vi "test-sync singleline loop.vi"(8 "error in (no error)":errorcluster, 11 "TestCase in":refnum<class "testcase-csm loop support.lvclass">) -> (0 "error out":errorcluster, 3 "TestCase out":refnum<class "testcase-csm loop support.lvclass">)   [LabVIEW 2017, in "testcase-csm loop support.lvclass"]
uses:
  testcase-csm loop support.lvclass
  56d4bdba-c2f1-4b55-add1-7a078de9da03.vi
  ea54eaf7-6c78-4206-8259-080cdfbb85de.vi
  src/user.lib/_NEVSTOP/Communicable State Machine(CSM)/AdvanceAPI/CSM - Revert Arguments-Safe String.vi
  src/user.lib/_NEVSTOP/Communicable State Machine(CSM)/_Shared/Trim Single-line Text.vi
  src/user.lib/_NEVSTOP/Communicable State Machine(CSM)/AdvanceAPI/CSM - Make String Arguments Safe.vi
  src/user.lib/_NEVSTOP/Communicable State Machine(CSM)/AdvanceAPI/CSM - Break Down Multiple States String.vi
  src/user.lib/_NEVSTOP/Communicable State Machine(CSM)/AdvanceAPI/CSM - Compact Multiple States.vi
  src/user.lib/_NEVSTOP/Communicable State Machine(CSM)/AdvanceAPI/CSM - Keywords.vi
  <vilib>/addons/_JKI Toolkits/VI Tester/TestCase.llb/TestCase.lvclass
  src/user.lib/_NEVSTOP/Communicable State Machine(CSM)/Communicable State Machine.lvlib
  src/user.lib/_NEVSTOP/Communicable State Machine(CSM)/addons/Loop-Support/CSM Loop Support.lvlib
  C:/Program Files (x86)/National Instruments/LabVIEW 2017/vi.lib/addons/_JKI Toolkits/VI Tester/TestCase.llb/TestCase.lvclass
panel:
  out "State History":string
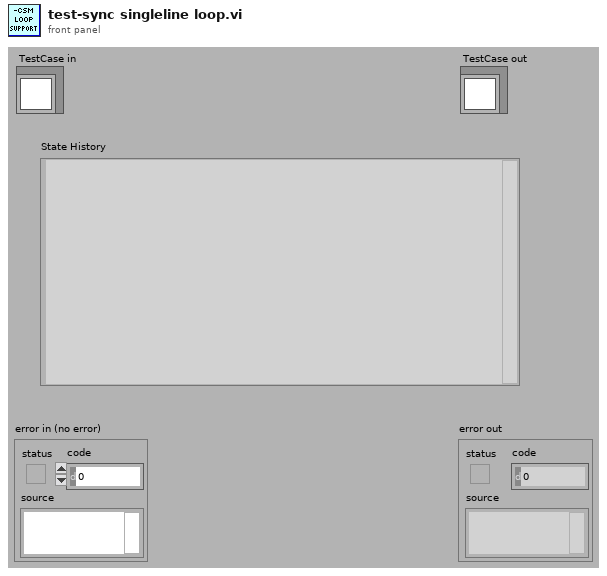
[diagram p1: front panel]
types:
  T1 = enum32{"Invalid", "Standard", "Closed", "Hidden", "Minimized", "Maximized"}
  T2 = enum32{"invalid app kind", "Development System", "Run Time System", "Student Edition", "Embedded LabVIEW", "Evaluation", "Custom"}
  T3 = typedef "Communicable State Machine.lvlib/_CSM_Response Source Message.ctl" = cluster{"‘State":string, "’Arguments":string, "’Error":errorcluster}
  T4 = cluster{"Current VI Reference":refnum<vi>, "Close Panel on Exit?":bool}
  T5 = cluster{"Core":cluster{"Current VI Reference":refnum<vi>, "Close Panel on Exit?":bool}, "diff":dbl, "time":timestamp}
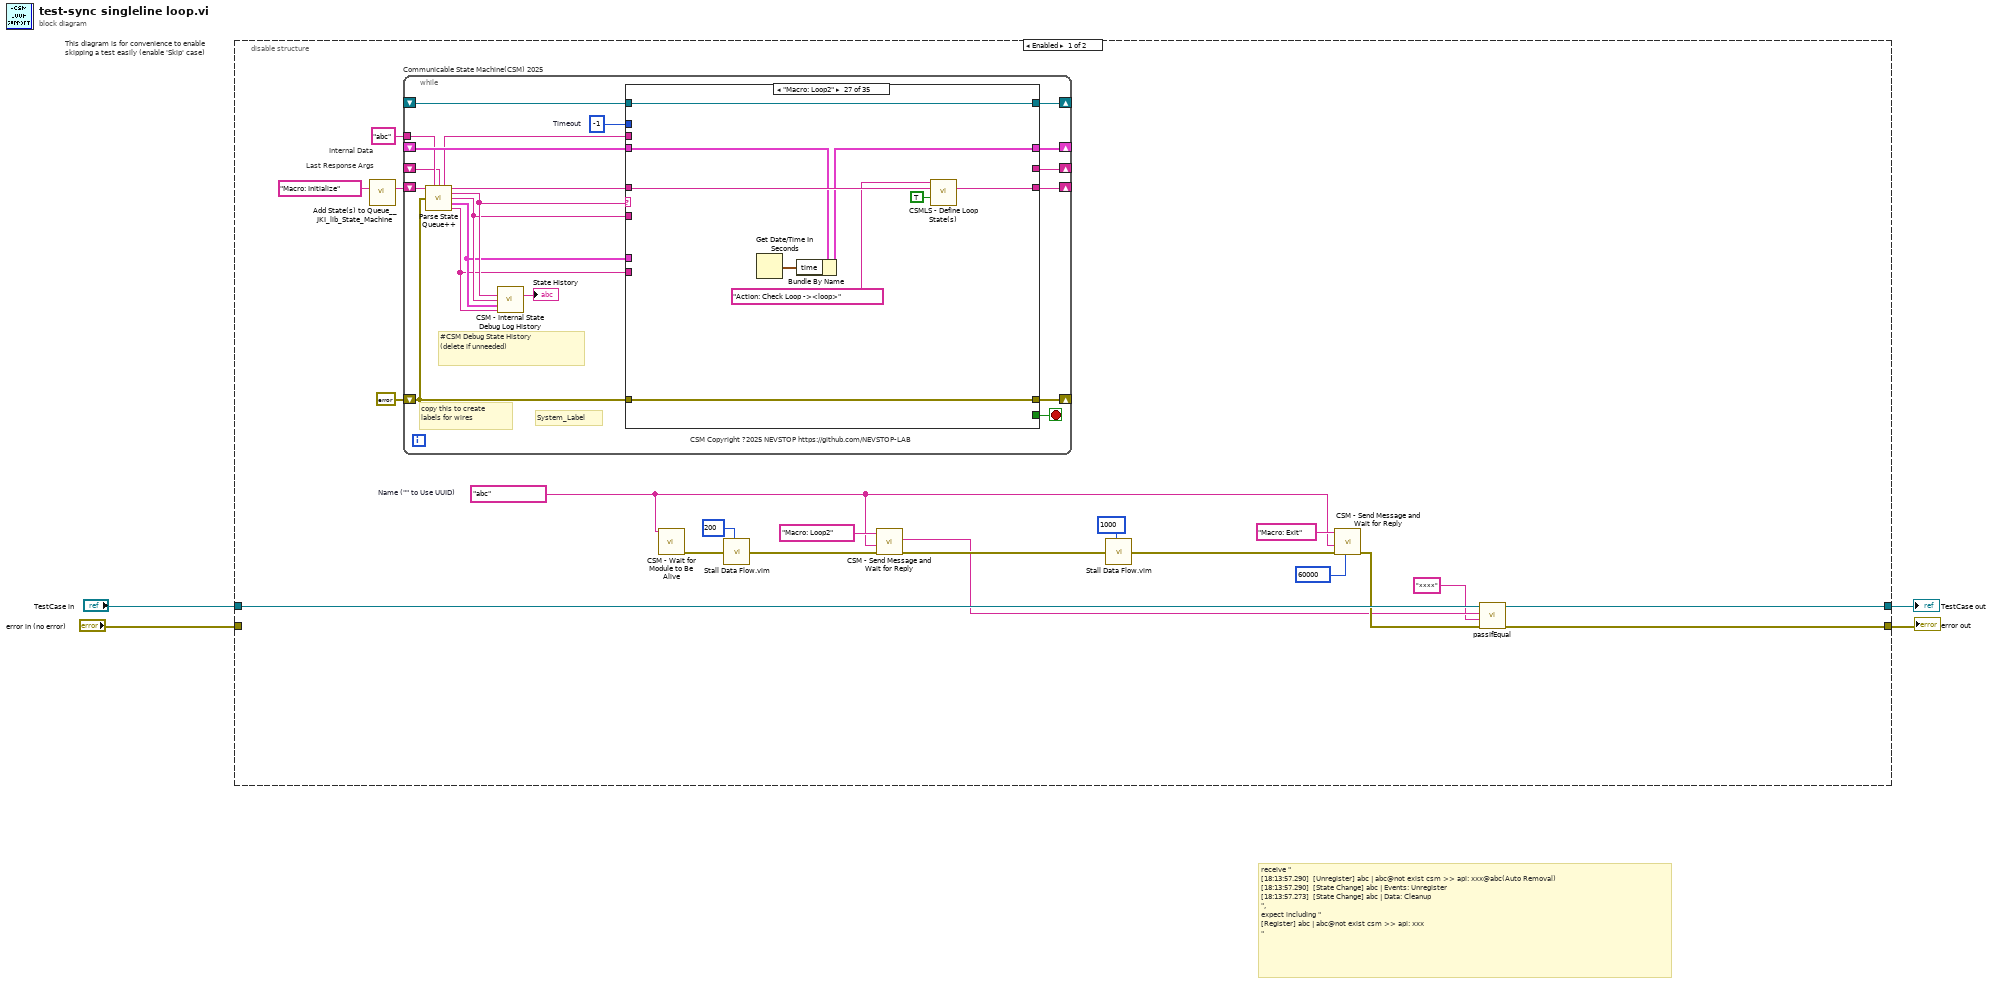
[diagram p0: block diagram]
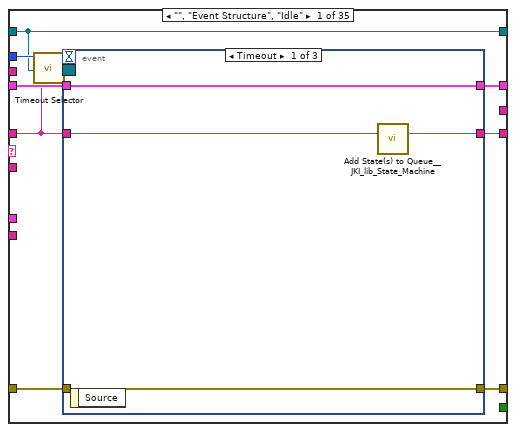
[diagram p2: hidden frame]
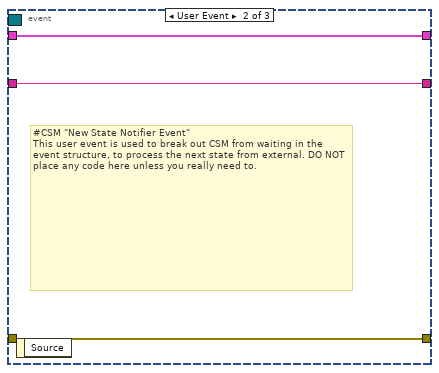
[diagram p3: hidden frame]
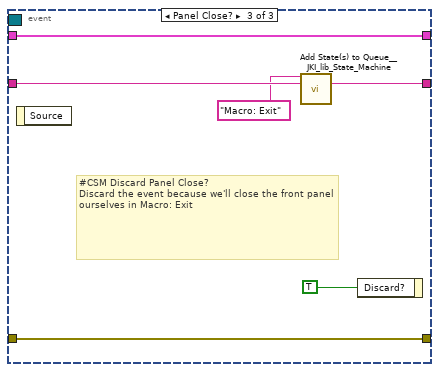
[diagram p4: hidden frame]
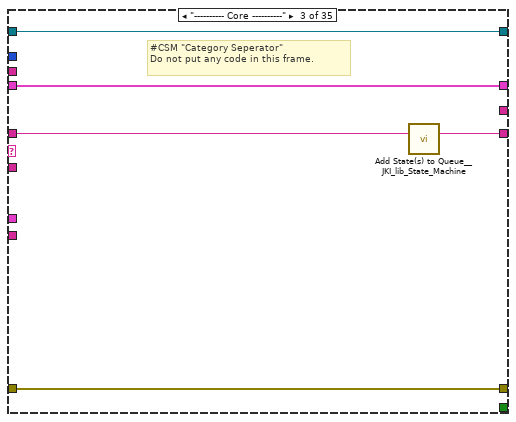
[diagram p6: hidden frame]
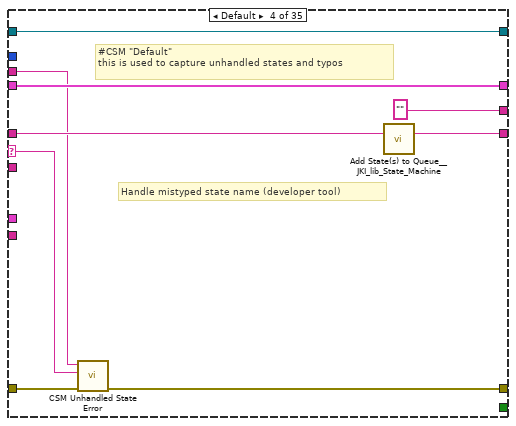
[diagram p7: hidden frame]
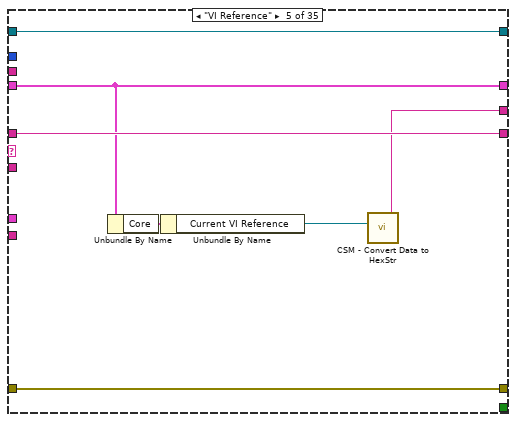
[diagram p8: hidden frame]
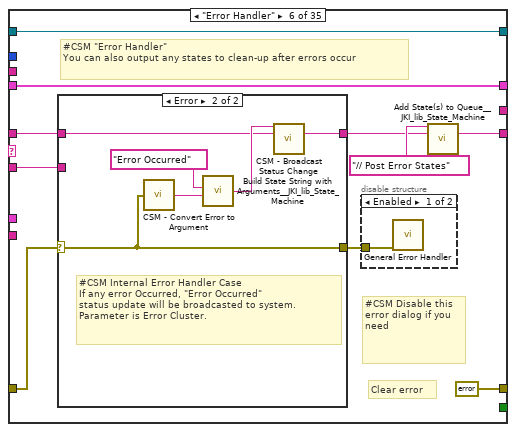
[diagram p9: hidden frame]
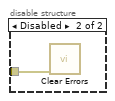
[diagram p10: hidden frame]
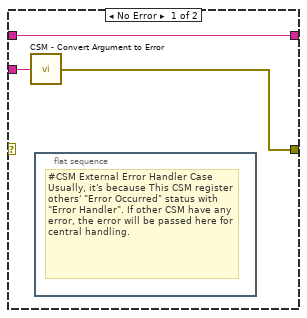
[diagram p11: hidden frame]
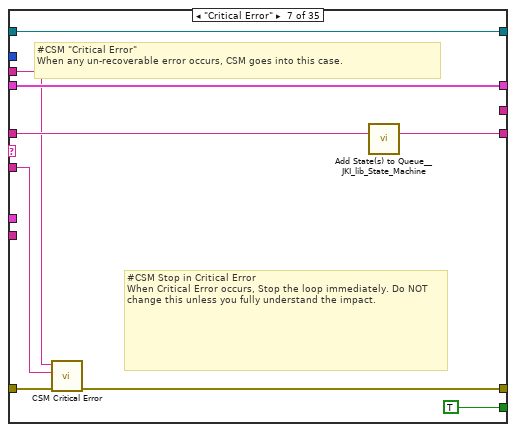
[diagram p12: hidden frame]
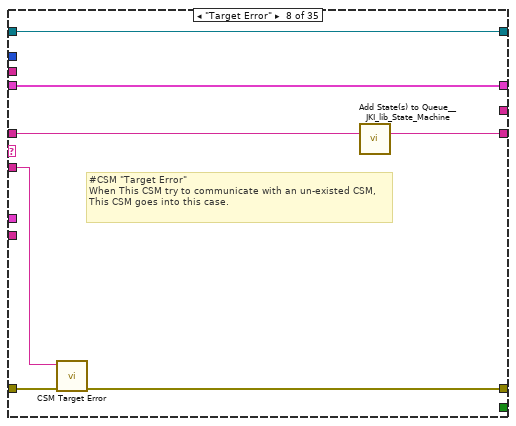
[diagram p13: hidden frame]
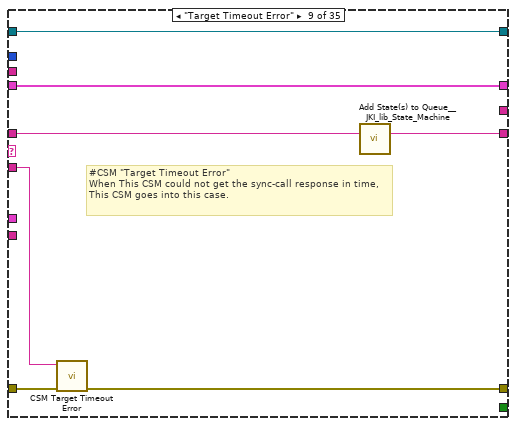
[diagram p14: hidden frame]
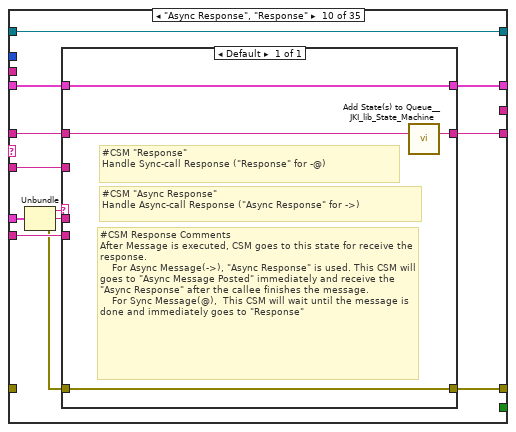
[diagram p15: hidden frame]
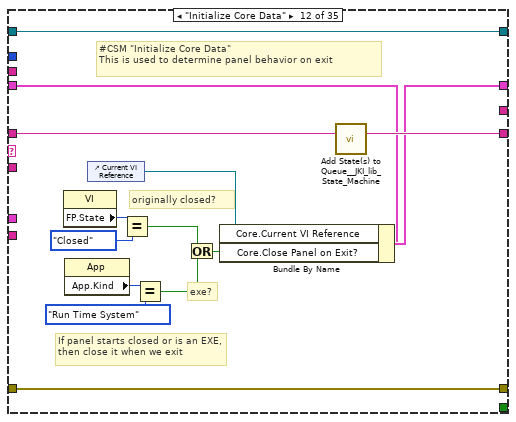
[diagram p17: hidden frame]
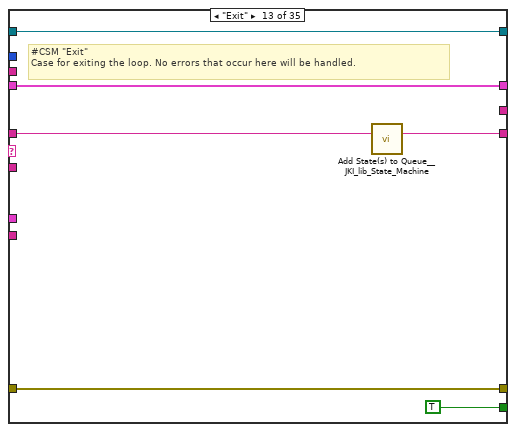
[diagram p18: hidden frame]
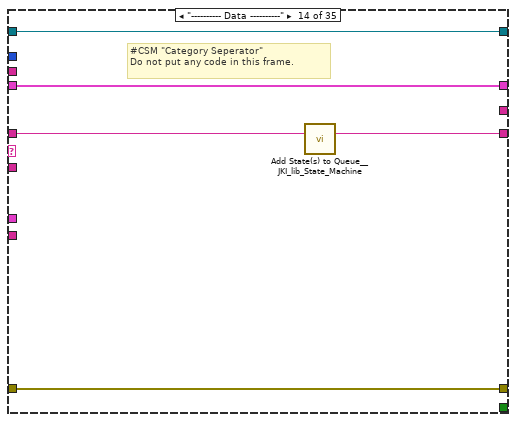
[diagram p19: hidden frame]
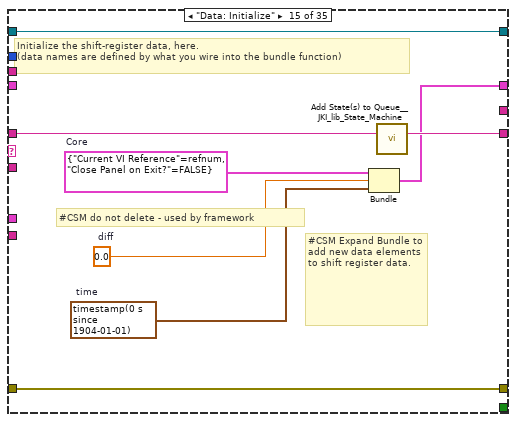
[diagram p20: hidden frame]
diagram:
  # "receive \"\n[18:13:57.290]  [Unregister] abc | abc@not exist csm >> api: xxx@abc(Auto Removal)\n[18:13:57.290]  [State Change] abc | Events: Unregister\n[18:13:57.273]  [State Change] abc | Data: Cleanup\n\", \nexpect including \"\n[Register] abc | abc@not exist csm >> api: xxx\n\""
  n1 = disable-structure "This diagram is for convenience to enable skipping a test easily (enable 'Skip' case)" shown="Enabled" {
    disable-tunnel: "TestCase in" -> [w15 w406]
    disable-tunnel: [w13 w404] -> w1
    disable-tunnel: [w12 w405] -> w3
    disable-tunnel: "error in (no error)" -> [_ w403]
    frame Enabled {
      w18 = "abc"  # Name ("" to Use UUID)
      # "Last Response Args"
      # "Internal Data"
      n2 = call <vilib>:"Add State(s) to Queue__JKI_lib_State_Machine.vi"("State(s) in (\"\")"="Macro: Initialize" ("Init State(\"Macro: Initialize\")")) -> ("States Out"=w22:string)  [unwired: 14 in]
      n3 = while "Communicable State Machine(CSM) 2025" {
        shift-right: [w39] -> _
        shift-left: _ -> [w38]
        shift-right: [w42] -> _
        shift-left: errorcluster {"status"=FALSE, "code"=0, "source"=""} ("error out") -> [w36]
        shift-right: [w41] -> _
        shift-left: w22 -> [w43]
        tunnel: "abc" ("Name (\"\" to Use UUID)") -> [w32]
        shift-right: [w35] -> _
        shift-left: _ -> [w26]
        shift-right: [w34] -> _
        shift-left: _ -> [w33]
        stop <- w40 stop-if-true
        w37 = -1  # Timeout
        # "#CSM Debug State History\n(delete if unneeded)"
        # "copy this to create labels for wires"
        # "System_Label"
        # "CSM Copyright ?2025 NEVSTOP https://github.com/NEVSTOP-LAB"
        n4 = call "Parse State Queue++.vi"("State Queue"=w43, "Name (\"\" to Use UUID)"=w32, "Response Arguments"=w26, "Previous Error"=w36) -> ("Name Used"=w27:string, "Remaining States"=w44:string, "Current State"=w31:string, "Arguments"=w30:string, "Additional Information"=w29:T3, "Source CSM"=w28:string)  [unwired: 6 in]
        n5 = call "CSM - Internal State Debug Log History.vi"("State"=w31, "Arguments (\"\")"=w30, ">> Response Source Message >>"=w29, "Source (\"\")"=w28) -> ("Debug Log"=→"State History":string)  [unwired: 11 in]
        n6 = case shown="\"Macro: Loop2\"" w31 {
          selector: w31 -> [_ _ _ w78 _ _ _ _ _ _ _ _ _ _ _ _ _ _ _ _ _ _ _ _ _ _ _ _ _ _ _ _ _ w388 _]
          tunnel: w44 -> [w45 w69 w75 w83 w90 w96 w119 w125 w132 w141 w154 w169 w175 w180 w188 w195 w200 w207 w211 w217 w222 w229 w245 w315 w321 w328 w337 w349 w352 w357 w363 w371 w378 w389 w401]
          tunnel: w30 -> [_ _ _ _ _ w95 w114 w124 w131 w140 _ _ _ _ _ _ _ _ _ _ _ w224 w239 _ _ _ _ _ _ _ w360 _ _ _ _]
          tunnel: w38 -> [w52 w68 w72 w81 w89 w100 w120 w127 w134 w143 w153 w162 w173 w177 _ w190 w197 w206 w210 w214 w220 w227 w241 w312 w318 w325 w334 w346 w351 w356 w362 w368 w375 w385 w399]
          tunnel: [w51 w70 w73 w76 w91 errorcluster {"status"=FALSE, "code"=0, "source"=""} ("error out") w115 w122 w129 w146 w155 w166 w172 w178 w185 w191 w198 w201 w209 w215 w219 w225 w242 w313 w319 w326 w335 w347 w353 w358 w364 w369 w376 w391 w402] -> w42
          tunnel: w36 -> [w50 w70 w73 w84 w91 w97 w121 w123 w130 _ w155 w166 w172 w178 w185 w192 w198 _ w212 w215 w219 w226 w243 w313 w319 w326 w335 w347 w353 w358 w364 w369 w376 w391 w402]
          tunnel: [w53 w69 w74 w82 w90 w92 w118 w128 w135 w142 w154 w168 w174 w179 w187 w194 w199 w207 w211 w216 w221 w228 w244 w314 w320 w327 w336 w348 w352 w357 w363 w370 w377 w392 w401] -> w41
          tunnel: [_ _ _ _ _ _ TRUE _ _ _ _ _ TRUE _ _ _ _ _ _ _ _ _ _ _ _ _ _ _ _ _ _ _ _ _ _] -> w40
          tunnel: [w49 w68 w72 w81 w89 w100 w120 w127 w134 w144 w153 w167 w173 w177 w186 w190 w197 w206 w210 w214 w220 w227 w241 w312 w318 w325 w331 w346 w351 w356 w362 w368 w373 w381 w399] -> w39
          tunnel: w37 -> [w48 _ _ _ _ _ _ _ _ _ _ _ _ _ _ _ _ _ _ _ _ _ _ _ _ _ _ _ _ _ _ _ _ _ _]
          tunnel: w28 -> [_ _ _ _ _ _ _ _ _ w138 _ _ _ _ _ _ _ _ _ _ _ _ _ _ _ _ _ _ _ _ _ _ _ _ _]
          tunnel: w29 -> [_ _ _ _ _ _ _ _ _ w145 _ _ _ _ _ _ _ _ _ _ _ _ _ _ _ _ _ _ _ _ _ _ _ _ _]
          tunnel: [_ _ _ "" w85 _ _ _ _ _ _ _ _ _ _ _ _ _ _ _ _ _ _ _ _ _ _ _ _ "API1 Response" w359 _ _ "xxxx" ("HEX String (0-9,A-F)") "Done" ("HEX String (0-9,A-F)")] -> w35
          tunnel: [w47 w67 w71 w79 w88 w99 w116 w126 w133 w147 w152 w156 w170 w176 w181 w189 w196 w205 w208 w213 w218 w223 w238 w311 w316 w323 w332 w339 w350 w355 w361 w367 w374 w390 w400] -> w34
          tunnel: w33 -> [w47 w67 w71 w79 w88 w99 w116 w126 w133 w147 w152 w156 w170 w176 w181 w189 w196 _ w208 w213 w218 w223 w238 w311 w316 w323 w332 w339 w350 w355 w361 w367 w374 w390 w400]
          tunnel: w27 -> [_ _ _ w77 _ _ w113 _ _ _ _ _ _ _ _ _ _ w204 _ _ _ _ _ _ _ _ _ _ _ _ _ _ _ _ _]
          frame "", "Event Structure", "Idle" {
            n7 = call "Timeout Selector.vi"("Remaining States"=w45, "Timeout Expected"=w48) -> ("Timeout"=w46:i32)  [unwired: 5 in]
            n8 = event shown="[0] Timeout" {
              selector: w47 -> [_ _ _]
              dyn-events: _ -> [_ _ _]
              timeout: w46 -> [_ _ _]
              tunnel: w45 -> [w57 w59 w66]
              tunnel: [w56 w59 w65] -> w53
              tunnel: w52 -> [w54 w60 w63]
              tunnel: [w55 w58 w64] -> w51
              tunnel: w50 -> [w55 w58 w64]
              tunnel: [w54 w60 w63] -> w49
              event Timeout {
                n9 = event-data() -> ()  [unwired: 1 in, 1 out]
                n10 = call <vilib>:"Add State(s) to Queue__JKI_lib_State_Machine.vi"("State(s) in (\"\")"=w57) -> ("States Out"=w56:string)  [unwired: 14 in]
              }
              event User Event {
                # "#CSM \"New State Notifier Event\"\nThis user event is used to break out CSM from waiting in the event structure, to process the next state from external. DO NOT place any code here unless you really need to."
                n11 = event-data() -> ()  [unwired: 1 in, 1 out]
              }
              event Panel Close? {
                # "#CSM Discard Panel Close?\nDiscard the event because we'll close the front panel ourselves in Macro: Exit"
                n12 = event-data() -> ()  [unwired: 1 in, 1 out]
                n13 = call <vilib>:"Add State(s) to Queue__JKI_lib_State_Machine.vi"("State(s) in Front (\"\")"="Macro: Exit", "State(s) in (\"\")"=w66) -> ("States Out"=w65:string)  [unwired: 13 in]
                n14 = event-data("Discard?"=TRUE) -> ()  [unwired: 1 in, 1 out]
              }
            }
          }
          frame "CSM Documentation" {
            # "#CSM README FIRST\n\nCommunicable State Machine(CSM) is a LabVIEW application framework that builds upon JKI State Machine(JKISM). It follows the pattern of JKISM and extends the keywords to describe message communication between modules, including concepts such as Sync-Message, Async-Message, Subscription/Unsubscription of status - essential elements for creating reusable code modules. For more information, please visit the CSM wiki: https://nevstop-lab.github.io/CSM-Wiki/\n\nFor instructions on JKI State Machine, visit: http://jki.net/state-machine/\nFor information about CSM, visit: https://github.com/NEVSTOP-LAB"
            # "#CSM \"Documentation\"\nCase for holding CSM Documenation"
          }
          frame "---------- Core ----------" {
            # "#CSM \"Category Seperator\"\nDo not put any code in this frame."
            n15 = call <vilib>:"Add State(s) to Queue__JKI_lib_State_Machine.vi"("State(s) in (\"\")"=w75) -> ("States Out"=w74:string)  [unwired: 14 in]
          }
          frame Default {
            # "#CSM \"Default\"\nthis is used to capture unhandled states and typos"
            # "Handle mistyped state name (developer tool)"
            n16 = call "CSM Unhandled State Error.vi"("error in (no error)"=w84, "Undefined State"=w78, "CSM Name"=w77) -> ("error out"=w76:errorcluster)  [unwired: 8 in]
            n17 = call <vilib>:"Add State(s) to Queue__JKI_lib_State_Machine.vi"("State(s) in (\"\")"=w83) -> ("States Out"=w82:string)  [unwired: 14 in]
          }
          frame "VI Reference" {
            n18 = Unbundle By Name(w89) -> ("Core"=w87:T4)
            n19 = Unbundle By Name(w87) -> ("Current VI Reference"=w86:refnum<vi>)
            n20 = call "CSM - Convert Data to HexStr.vi"("Variant"=w86) -> ("HEX String (0-9,A-F)"=w85:string)  [unwired: 8 in]
          }
          frame "Error Handler" {
            # "#CSM Disable this error dialog if you need"
            # "#CSM \"Error Handler\"\nYou can also output any states to clean-up after errors occur"
            # "Clear error"
            n21 = case shown="Error" w97 {
              selector: w97 -> [_ w107]
              tunnel: [w106 w109] -> w93
              tunnel: w96 -> [w106 w108]
              tunnel: w95 -> [w105 _]
              tunnel: [w104 w107] -> w98
              frame No Error {
                n22 = call "CSM - Convert Argument to Error.vi"("Argument"=w105) -> ("Error"=w104:errorcluster)  [unwired: 4 in]
                n23 = flat-sequence {
                  frame #0 {
                    # "#CSM External Error Handler Case\nUsually, it's because This CSM register others' \"Error Occurred\" status with \"Error Handler\". If other CSM have any error, the error will be passed here for central handling."
                  }
                }
              }
              frame Error {
                # "#CSM Internal Error Handler Case \nIf any error Occurred, \"Error Occurred\" \nstatus update will be broadcasted to system.\nParameter is Error Cluster."
                n24 = call "CSM - Convert Error to Argument.vi"("Error"=w107) -> ("Argument"=w111:string)  [unwired: 4 in]
                n25 = call <vilib>:"Build State String with Arguments__JKI_lib_State_Machine.vi"("Arguments (\"\")"=w111, "State"="Error Occurred" ("Status with Arguments")) -> ("State with Arguments"=w110:string)  [unwired: 4 in]
                n26 = call "CSM - Broadcast Status Change.vi"("Status With Arguments"=w110, "State Queue"=w108) -> ("Remaining States"=w109:string)  [unwired: 13 in]
              }
            }
            n27 = disable-structure shown="Enabled" {
              disable-tunnel: w98 -> [w102 w103]
              frame Enabled {
                n28 = call <vilib>:"General Error Handler.vi"("error in (no error)"=w102) -> ()  [unwired: 10 in, 5 out]
              }
              frame Disabled {
                n29 = call <vilib>:"Clear Errors.vi"("error in (no error)"=w103) -> ()  [unwired: 5 in, 2 out]
              }
            }
            n30 = call <vilib>:"Add State(s) to Queue__JKI_lib_State_Machine.vi"("State(s) in Front (\"\")"="// Post Error States", "State(s) in (\"\")"=w93) -> ("States Out"=w92:string)  [unwired: 13 in]
          }
          frame "Critical Error" {
            # "#CSM Stop in Critical Error\nWhen Critical Error occurs, Stop the loop immediately. Do NOT change this unless you fully understand the impact."
            # "#CSM \"Critical Error\"\nWhen any un-recoverable error occurs, CSM goes into this case."
            n31 = call "CSM Critical Error.vi"("error in (no error)"=w121, "Arugments (As Reason)"=w114, "CSM Name"=w113) -> ("error out"=w115:errorcluster)  [unwired: 8 in]
            n32 = call <vilib>:"Add State(s) to Queue__JKI_lib_State_Machine.vi"("State(s) in (\"\")"=w119) -> ("States Out"=w118:string)  [unwired: 14 in]
          }
          frame "Target Error" {
            # "#CSM \"Target Error\"\nWhen This CSM try to communicate with an un-existed CSM, This CSM goes into this case."
            n33 = call "CSM Target Error.vi"("error in (no error)"=w123, "Arguments (As CSM Name)"=w124) -> ("error out"=w122:errorcluster)  [unwired: 9 in]
            n34 = call <vilib>:"Add State(s) to Queue__JKI_lib_State_Machine.vi"("State(s) in (\"\")"=w125) -> ("States Out"=w128:string)  [unwired: 14 in]
          }
          frame "Target Timeout Error" {
            # "#CSM \"Target Timeout Error\"\nWhen This CSM could not get the sync-call response in time, This CSM goes into this case."
            n35 = call "CSM Target Timeout Error.vi"("error in (no error)"=w130, "Arguments (As CSM Name)"=w131) -> ("error out"=w129:errorcluster)  [unwired: 9 in]
            n36 = call <vilib>:"Add State(s) to Queue__JKI_lib_State_Machine.vi"("State(s) in (\"\")"=w132) -> ("States Out"=w135:string)  [unwired: 14 in]
          }
          frame "Async Response", "Response" {
            n37 = Unbundle(w145) -> ("‘State"=w139:string, "’Arguments"=w137:string, "’Error"=w136:errorcluster)
            n38 = case shown="Default" w139 {
              tunnel: [w151] -> w146
              tunnel: w136 -> [w151]
              tunnel: [w150] -> w144
              tunnel: w143 -> [w150]
              tunnel: [w148] -> w142
              tunnel: w141 -> [w149]
              tunnel: w140 -> [_]
              tunnel: w138 -> [_]
              tunnel: w137 -> [_]
              frame Default {
                # "#CSM Response Comments\nAfter Message is executed, CSM goes to this state for receive the response.\n    For Async Message(->), \"Async Response\" is used. This CSM will goes to \"Async Message Posted\" immediately and receive the \"Async Response\" after the callee finishes the message.\n    For Sync Message(@),  This CSM will wait until the message is done and immediately goes to \"Response\""
                # "#CSM \"Async Response\"\nHandle Async-call Response (\"Async Response\" for ->)"
                # "#CSM \"Response\"\nHandle Sync-call Response (\"Response\" for -@)"
                n39 = call <vilib>:"Add State(s) to Queue__JKI_lib_State_Machine.vi"("State(s) in (\"\")"=w149) -> ("States Out"=w148:string)  [unwired: 14 in]
              }
            }
          }
          frame "Async Message Posted" {
            # "#CSM \"Async Message Posted\"\nAfter Async Message is posted (-> or ->| ), CSM goes to this state for post-action.\nYou can use Argument - State to tell which Async Message is called."
          }
          frame "Initialize Core Data" {
            # "#CSM \"Initialize Core Data\"\nThis is used to determine panel behavior on exit"
            # "originally closed?"
            # "exe?"
            # "If panel starts closed or is an EXE, then close it when we exit"
            n40 = property class="VI"() -> ("FP.State"=w159:T1)  [unwired: 2 in, 2 out]
            n41 = property class="App"() -> ("App.Kind"=w165:T2)  [unwired: 2 in, 2 out]
            n42 = control-ref of="Current VI Reference"() -> (w160:refnum<vi>)
            n43 = Equal?(x=w159, y=T1."Closed" ("Front Panel Window:State")) -> (x = y?=w157:bool)
            n44 = Equal?(x=w165, y=T2."Run Time System" ("Application:Kind")) -> (x = y?=w163:bool)
            n45 = Or(x=w157, y=w163) -> (x .or. y?=w161:bool)
            n46 = Bundle By Name(cluster=w162, "Core.Current VI Reference"=w160, "Core.Close Panel on Exit?"=w161) -> (w167:T5)
            n47 = call <vilib>:"Add State(s) to Queue__JKI_lib_State_Machine.vi"("State(s) in (\"\")"=w169) -> ("States Out"=w168:string)  [unwired: 14 in]
          }
          frame "Exit" {
            # "#CSM \"Exit\"\nCase for exiting the loop. No errors that occur here will be handled."
            n48 = call <vilib>:"Add State(s) to Queue__JKI_lib_State_Machine.vi"("State(s) in (\"\")"=w175) -> ("States Out"=w174:string)  [unwired: 14 in]
          }
          frame "---------- Data ----------" {
            # "#CSM \"Category Seperator\"\nDo not put any code in this frame."
            n49 = call <vilib>:"Add State(s) to Queue__JKI_lib_State_Machine.vi"("State(s) in (\"\")"=w180) -> ("States Out"=w179:string)  [unwired: 14 in]
          }
          frame "Data: Initialize" {
            w182 = T4 {"Current VI Reference"=refnum, "Close Panel on Exit?"=FALSE}  # Core
            w184 = 0.0  # diff
            w183 = timestamp(0 s since 1904-01-01)  # time
            # "#CSM do not delete - used by framework"
            # "#CSM Expand Bundle to add new data elements to shift register data."
            # "Initialize the shift-register data, here.\n(data names are defined by what you wire into the bundle function)"
            n50 = Bundle("Core"=w182, "diff"=w184, "time"=w183) -> (w186:T5)  [unwired: 1 in]
            n51 = call <vilib>:"Add State(s) to Queue__JKI_lib_State_Machine.vi"("State(s) in (\"\")"=w188) -> ("States Out"=w187:string)  [unwired: 14 in]
          }
          frame "Data: Cleanup" {
            # "Cleanup any data and references, here.\n(this is called automatically, by the Macro: Exit)"
            n52 = Unbundle By Name(w190) -> ("Core.Current VI Reference"=w193:refnum<vi>)
            n53 = Close Reference(reference=w193, error in (no error)=w192) -> (error out=w191:errorcluster)
            n54 = call <vilib>:"Add State(s) to Queue__JKI_lib_State_Machine.vi"("State(s) in (\"\")"=w195) -> ("States Out"=w194:string)  [unwired: 14 in]
          }
          frame "---------- Events ----------" {
            # "#CSM \"Category Seperator\"\nDo not put any code in this frame."
            n55 = call <vilib>:"Add State(s) to Queue__JKI_lib_State_Machine.vi"("State(s) in (\"\")"=w200) -> ("States Out"=w199:string)  [unwired: 14 in]
          }
          frame "Events: Register" {
            # "#CSM \"Events: Register\"\nRegister user event. New Message Event is registered to break CSM waiting in event structure by default."
            # "#CSM Register New Message Event\nRegister message event to break Waiting in Event structure."
            n56 = call "CSM - Get New State Notifier Event.vi"("Name (\"\" to Use UUID)"=w204) -> ("error out"=w202:errorcluster, "New State Notifier Event"=w203:refnum<user-event>)  [unwired: 9 in]
            n57 = register-events(error in=w202, w203) -> (reference out=w205:refnum<event-registration>, error out=w201:errorcluster)  [unwired: 1 in]
          }
          frame "Events: Unregister" {
            # "#CSM \"Events: Unregister\"\nUnregister user event."
            n58 = Unregister For Events(event registration refnum=w208, error in=w212) -> (error out=w209:errorcluster)
          }
          frame "---------- UI ----------" {
            # "#CSM \"Category Seperator\"\nDo not put any code in this frame."
            n59 = call <vilib>:"Add State(s) to Queue__JKI_lib_State_Machine.vi"("State(s) in (\"\")"=w217) -> ("States Out"=w216:string)  [unwired: 14 in]
          }
          frame "UI: Initialize" {
            # "#CSM \"UI: Initialize\"\nInitialize the User Interface, here.\n(this is called automatically, by the Macro: Init)"
            n60 = call <vilib>:"Add State(s) to Queue__JKI_lib_State_Machine.vi"("State(s) in (\"\")"=w222) -> ("States Out"=w221:string)  [unwired: 14 in]
          }
          frame "UI: Cursor Set" {
            # "#CSM \"UI: Cursor Set\"\nSet and Unset Cursor Busy.\n(Usage: \"UI: Cursor Set >> Busy|Idle\")"
            # "Argument"
            n61 = disable-structure shown="Default" {
              disable-tunnel: w226 -> [w232 w237]
              disable-tunnel: [w231 w237] -> w225
              disable-tunnel: w224 -> [w230 _]
              frame condition #0 (active) {
                n62 = case shown="\"Idle\", Default" w230 {
                  tunnel: w232 -> [w234 w236]
                  tunnel: [w233 w235] -> w231
                  frame "Idle", Default {
                    n63 = call <vilib>:"Unset Busy.vi"("error in (no error)"=w234) -> ("error out"=w233:errorcluster)  [unwired: 10 in]
                  }
                  frame "Busy" {
                    n64 = call <vilib>:"Set Busy.vi"("error in (no error)"=w236) -> ("error out"=w235:errorcluster)  [unwired: 9 in, 1 out]
                  }
                }
              }
              frame condition #1 {
              }
            }
            n65 = call <vilib>:"Add State(s) to Queue__JKI_lib_State_Machine.vi"("State(s) in (\"\")"=w229) -> ("States Out"=w228:string)  [unwired: 14 in]
          }
          frame "UI: Front Panel State" {
            # "#CSM \"UI: Front Panel State\"\nSet Front Panel Open or Closed\n(Usage: \"UI: Front Panel State >> Open|Close\")"
            # "Argument"
            n66 = Unbundle By Name(w241) -> ("Core.Current VI Reference"=w240:refnum<vi>)
            n67 = call <vilib>:"Add State(s) to Queue__JKI_lib_State_Machine.vi"("State(s) in (\"\")"=w245) -> ("States Out"=w244:string)  [unwired: 14 in]
            n68 = case shown="\"Close\", \"Closed\"" w239 {
              tunnel: w243 -> [w251 w266 w277 w290 w303]
              tunnel: [w253 w267 w279 w292 w305] -> w242
              tunnel: w240 -> [w252 w264 w278 w291 w304]
              frame "Open", "Standard", Default {
                w246 = T1."Standard" ("State")
                n69 = property class="VI"(reference=w252, error in=w251) -> (reference out=w249:refnum<vi>, error out=w250:errorcluster, "FP.State"=w248:T1)
                n70 = Not Equal?(x=w248, y=w246) -> (x != y?=w247:bool)
                n71 = case shown="True" w247 {
                  tunnel: [w257 w259] -> w253
                  tunnel: w250 -> [w256 w259]
                  tunnel: w249 -> [w255 _]
                  tunnel: w246 -> [w254 _]
                  frame True {
                    n72 = invoke class="VI" method="FP.Open"(reference=w255, error in=w256, "Activate"=TRUE, "State"=w254) -> (error out=w257:errorcluster)  [unwired: 1 in, 4 out]
                  }
                  frame False {
                  }
                }
              }
              frame "Close", "Closed" {
                n73 = property class="VI"(reference=w264, error in=w266) -> (reference out=w263:refnum<vi>, error out=w265:errorcluster, "FP.State"=w261:T1)
                n74 = Not Equal?(x=w261, y=T1."Closed" ("Front Panel Window:State")) -> (x != y?=w260:bool)
                n75 = case shown="False" w260 {
                  tunnel: [w268 w271] -> w267
                  tunnel: w265 -> [w268 w270]
                  tunnel: w263 -> [_ w269]
                  frame False {
                  }
                  frame True {
                    n76 = invoke class="VI" method="FP.Close"(reference=w269, error in=w270) -> (error out=w271:errorcluster)  [unwired: 1 in, 2 out]
                  }
                }
              }
              frame "Hidden", "Hide" {
                w272 = T1."Hidden" ("State")
                n77 = property class="VI"(reference=w278, error in=w277) -> (reference out=w275:refnum<vi>, error out=w276:errorcluster, "FP.State"=w274:T1)
                n78 = Not Equal?(x=w274, y=w272) -> (x != y?=w273:bool)
                n79 = case shown="True" w273 {
                  tunnel: [w283 w284] -> w279
                  tunnel: w276 -> [w282 w284]
                  tunnel: w275 -> [w281 _]
                  tunnel: w272 -> [w280 _]
                  frame True {
                    n80 = invoke class="VI" method="FP.Open"(reference=w281, error in=w282, "State"=w280) -> (error out=w283:errorcluster)  [unwired: 2 in, 4 out]
                  }
                  frame False {
                  }
                }
              }
              frame "Minimize", "Minimized" {
                w285 = T1."Minimized" ("State")
                n81 = property class="VI"(reference=w291, error in=w290) -> (reference out=w288:refnum<vi>, error out=w289:errorcluster, "FP.State"=w287:T1)
                n82 = Not Equal?(x=w287, y=w285) -> (x != y?=w286:bool)
                n83 = case shown="True" w286 {
                  tunnel: [w296 w297] -> w292
                  tunnel: w289 -> [w295 w297]
                  tunnel: w288 -> [w294 _]
                  tunnel: w285 -> [w293 _]
                  frame True {
                    n84 = invoke class="VI" method="FP.Open"(reference=w294, error in=w295, "State"=w293) -> (error out=w296:errorcluster)  [unwired: 2 in, 4 out]
                  }
                  frame False {
                  }
                }
              }
              frame "Maximize", "Maximized" {
                w298 = T1."Maximized" ("State")
                n85 = property class="VI"(reference=w304, error in=w303) -> (reference out=w301:refnum<vi>, error out=w302:errorcluster, "FP.State"=w300:T1)
                n86 = Not Equal?(x=w300, y=w298) -> (x != y?=w299:bool)
                n87 = case shown="True" w299 {
                  tunnel: [w309 w310] -> w305
                  tunnel: w302 -> [w308 w310]
                  tunnel: w301 -> [w307 _]
                  tunnel: w298 -> [w306 _]
                  frame True {
                    n88 = invoke class="VI" method="FP.Open"(reference=w307, error in=w308, "State"=w306) -> (error out=w309:errorcluster)  [unwired: 2 in, 4 out]
                  }
                  frame False {
                  }
                }
              }
            }
          }
          frame "---------- Macro ----------" {
            # "#CSM \"Category Seperator\"\nDo not put any code in this frame."
            n89 = call <vilib>:"Add State(s) to Queue__JKI_lib_State_Machine.vi"("State(s) in (\"\")"=w315) -> ("States Out"=w314:string)  [unwired: 14 in]
          }
          frame "Macro: Initialize" {
            w317 = "Data: Initialize\nInitialize Core Data\nEvents: Register\nUI: Initialize\nUI: Front Panel State >> Open"  # Data: Initialize Initialize Core Data Events: Register UI: Initialize UI: Front Panel State >> Open
            # "#CSM \"Macro: Initialize\"\nInitialization Macro (This is called once, when the VI starts)"
            n90 = call <vilib>:"Add State(s) to Queue__JKI_lib_State_Machine.vi"("State(s) in Front (\"\")"=w317, "State(s) in (\"\")"=w321) -> ("States Out"=w320:string)  [unwired: 13 in]
          }
          frame "Macro: Loop" {
            n91 = call "CSMLS - Define Loop State(s).vi"("Loop States"="Action: Go\nAction: Check Loop -><loop>\nAction Return", "States Queue"=w328, "Add to Front? (F)"=TRUE ("Front(T)/Back(F)")) -> ("Remaining States"=w327:string)  [unwired: 12 in]
          }
          frame "Macro: Loop2" {
            n92 = Get Date/Time In Seconds() -> (seconds since 1Jan1904=w330:timestamp)
            n93 = Bundle By Name(cluster=w334, "time"=w330) -> (w331:T5)
            n94 = call "CSMLS - Define Loop State(s).vi"("Loop States"="Action: Check Loop -><loop>", "States Queue"=w337, "Add to Front? (F)"=TRUE ("Front(T)/Back(F)")) -> ("Remaining States"=w336:string)  [unwired: 12 in]
          }
          frame "Macro: Exit" {
            # "#CSM \"Macro: Exit\"\nExit Macro (This is called once, when the VI exits)"
            n95 = Unbundle By Name(w346) -> ("Core.Close Panel on Exit?"=w345:bool)
            n96 = Select(t="UI: Front Panel State >> Close", s=w345, f="") -> (s? t:f=w342:string)
            n97 = call <vilib>:"Add State(s) to Queue__JKI_lib_State_Machine.vi"("State(s) in Front (\"\")"="//Exit Sub-Modules ", "State(s) in (\"\")"=w342, "State(s) at Back (\"\")"="Data: Cleanup\nEvents: Unregister\nExit") -> ("States Out"=w340:string)  [unwired: 12 in]
            n98 = call <vilib>:"Add State(s) to Queue__JKI_lib_State_Machine.vi"("State(s) in Front (\"\")"=w340, "State(s) in (\"\")"=w349) -> ("States Out"=w348:string)  [unwired: 13 in]
          }
          frame "---------- API ----------" {
            # "#CSM \"Category Seperator\"\nDo not put any code in this frame."
          }
          frame "API: API1" {
            # "#CSM API Example\nCopy/Rename this case for your own API"
            # "#CSM Response\nConnect this to return the response of your API"
            # "#CSM >> Source CSM >>\nIf you need to tell who triggered this state , use this string. If it's this case itself, this string is \"\"."
            # "#CSM >> Arguments >>\nDeal with the parameter if any"
          }
          frame "API: API2" {
            # "#CSM API Example\nCopy/Rename this case for your own API"
            # "unpack Hex String  to Variant\nif complex parameter is needed."
            n99 = call "CSM - Convert HexStr to Data.vi"("HEX String"=w360) -> ()  [unwired: 7 in, 2 out]
            n100 = disable-structure shown="Disabled" {
              disable-tunnel: [w365 "API2 Response"] -> w359
              frame Disabled {
                # "pack variant to hexstr \nif complex response is needed."
                # "complex Response"
                n101 = call "CSM - Convert Data to HexStr.vi"() -> ("HEX String (0-9,A-F)"=w365:string)  [unwired: 9 in]
              }
              frame Enabled {
              }
            }
          }
          frame "---------- Action ----------" {
            # "#CSM \"Category Seperator\"\nDo not put any code in this frame."
            n102 = call <vilib>:"Add State(s) to Queue__JKI_lib_State_Machine.vi"("State(s) in (\"\")"=w371) -> ("States Out"=w370:string)  [unwired: 14 in]
          }
          frame "Action: Go" {
            n103 = Get Date/Time In Seconds() -> (seconds since 1Jan1904=w372:timestamp)
            n104 = Bundle By Name(cluster=w375, "time"=w372) -> (w373:T5)
            n105 = call <vilib>:"Add State(s) to Queue__JKI_lib_State_Machine.vi"("State(s) in (\"\")"=w378) -> ("States Out"=w377:string)  [unwired: 14 in]
          }
          frame "Action: Check Loop" {
            n106 = Unbundle By Name(w385) -> ("time"=w384:timestamp)
            n107 = Wait (ms)(milliseconds to wait=u32 100) -> ()  [unwired: 1 out]
            n108 = Get Date/Time In Seconds() -> (seconds since 1Jan1904=w386:timestamp)
            n109 = Subtract(x=w386, y=w384) -> (x-y=w380:dbl)
            n110 = Greater?(x=w380, y=3.0) -> (0:w382:bool)
            n111 = case shown="True" w382 {
              tunnel: [w396 w397] -> w392
              tunnel: w389 -> [w395 w397]
              tunnel: w388 -> [w394 _]
              frame False {
                n112 = call "CSMLS - Append Continuous State.vi"("Loop State(s) And Arguments"="" ("Loop State(s) and Arguments"), "Continous State"=w394, "States Queue"=w395) -> ("Remaining States"=w396:string)  [unwired: 8 in]
              }
              frame True {
              }
            }
            n113 = Bundle By Name(cluster=w385, "diff"=w380) -> (w381:T5)
          }
          frame "Action Return" {
          }
        }
      }
      n114 = call "CSM - Wait for Module to Be Alive.vi"("CSM Name"=w18) -> ("error out"=w17:errorcluster)  [unwired: 12 in, 2 out]
      n115 = call "Stall Data Flow.vim"("value in"=w17, "milliseconds to wait"=u32 200) -> ("value out"=w7:errorcluster)  [unwired: 1 out]
      n116 = call "CSM - Send Message and Wait for Reply.vi"("Error In (No Error)"=w7, "Target Module"=w18, "State"="Macro: Loop2") -> ("error out"=w16:errorcluster, "Response"=w11:string)  [unwired: 6 in, 1 out]
      n117 = call "Stall Data Flow.vim"("value in"=w16, "milliseconds to wait"=u32 1000) -> ("value out"=w9:errorcluster)  [unwired: 1 out]
      n118 = call "CSM - Send Message and Wait for Reply.vi"("Response Timeout (-2 Using Global Settings)"=60000, "Error In (No Error)"=w9, "Target Module"=w18, "State"="Macro: Exit") -> ("error out"=w14:errorcluster)  [unwired: 5 in, 2 out]
      n119 = call-dynamic "passIfEqual.vi"("error in (no error)"=w14, "y"="xxxx" ("HEX String (0-9,A-F)"), "x"=w11, "TestCase in"=w15) -> ("error out"=w12:errorcluster, "TestCase out"=w13:refnum<class "testcase-csm loop support.lvclass">)  [unwired: 6 in]
    }
    frame Disabled {
      # "skip test result while test is under development"
      n120 = call <vilib>:"skip.vi"("error in (no error)"=w403, "TestCase in"=w406) -> ("error out"=w405:errorcluster, "TestCase out"=w404:refnum<class "testcase-csm loop support.lvclass">)  [unwired: 8 in]
    }
  }
  "error out" <- w3
  "TestCase out" <- w1
